vi "UMB_GTFO.vi"(10 "behavior weights":i8[](array[numeric])=[0, 1, 0], 11 "IR distance":dbl) -> (3 "Behavior Output":T1)   [LabVIEW 2012]
uses:
  NINJA Code/Tugboat/Robo_Programs/behaviorOutput_t.ctl
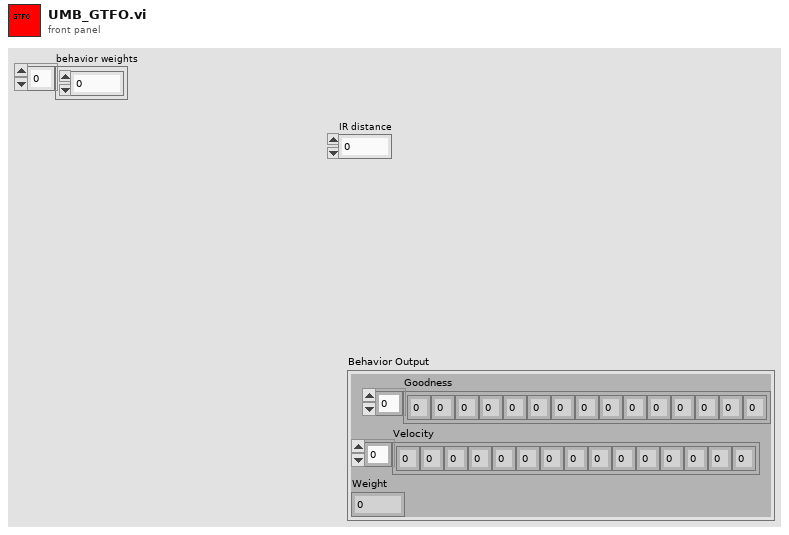
[diagram p1: front panel]
types:
  T1 = typedef "behaviorOutput_t.ctl" = cluster{"Goodness":i8[], "Velocity":i8[], "Weight":i8}
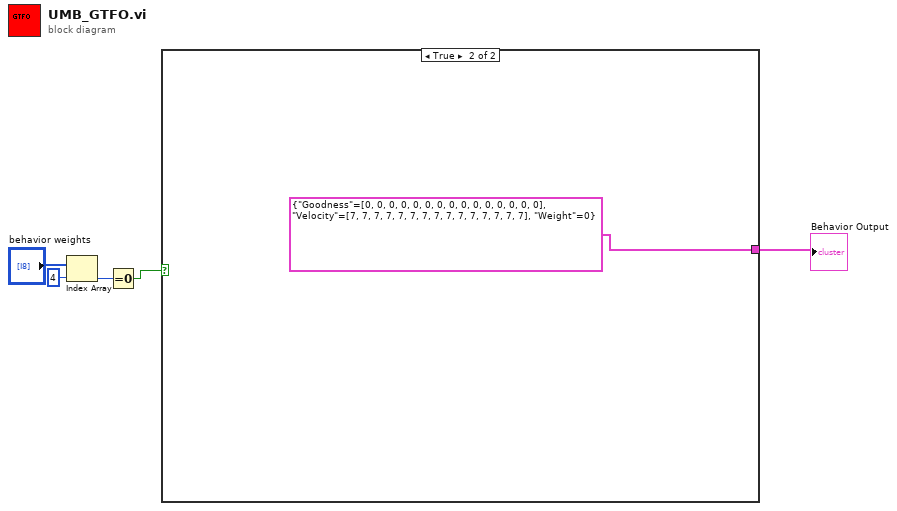
[diagram p0: block diagram]
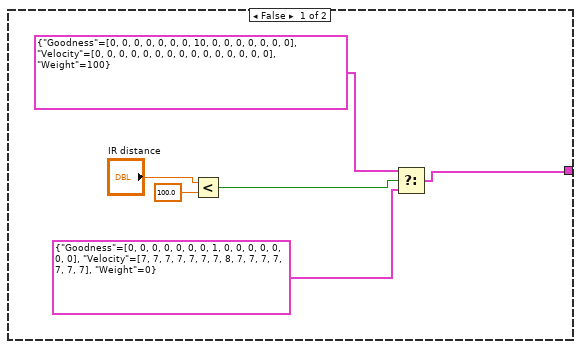
[diagram p2: hidden frame]
diagram:
  n1 = Index Array(array="behavior weights", index=4) -> (element=w4:i8)
  n2 = Equal To 0?(x=w4) -> (x = 0?=w5:bool)
  n3 = case shown="True" w5 {
    tunnel: [w6 T1 {"Goodness"=[0, 0, 0, 0, 0, 0, 0, 0, 0, 0, 0, 0, 0, 0, 0], "Velocity"=[7, 7, 7, 7, 7, 7, 7, 7, 7, 7, 7, 7, 7, 7, 7], "Weight"=0} ("Behavior Output")] -> w1
    frame False {
      n4 = Less?(x="IR distance", y=100.0) -> (x < y?=w7:bool)
      n5 = Select(t=T1 {"Goodness"=[0, 0, 0, 0, 0, 0, 0, 10, 0, 0, 0, 0, 0, 0, 0], "Velocity"=[0, 0, 0, 0, 0, 0, 0, 0, 0, 0, 0, 0, 0, 0, 0], "Weight"=100} ("Behavior Output"), s=w7, f=T1 {"Goodness"=[0, 0, 0, 0, 0, 0, 0, 1, 0, 0, 0, 0, 0, 0, 0], "Velocity"=[7, 7, 7, 7, 7, 7, 7, 8, 7, 7, 7, 7, 7, 7, 7], "Weight"=0} ("Behavior Output")) -> (s? t:f=w6:T1)
    }
    frame True {
    }
  }
  "Behavior Output" <- w1
